vi "Img_Center_Crop.vi"(7 "Crop_CFG":T2, 8 "error in":errorcluster, 9 "Image Dest In":T1, 11 "Image Src In":T1) -> (0 "error out":errorcluster, 3 "Image Dest Out":T1)   [LabVIEW 2020]
uses:
  <vilib>/vision/Image Controls.llb/IMAQ Image.ctl
  <vilib>/Ngene/DeepLTK Anomaly Detection Addon/Toolkit/API/Controls/Crop_CFG.ctl
  <vilib>/vision/NI_Vision_Development_Module.lvlib
  <vilib>/Ngene/DeepLTK Anomaly Detection Addon/Toolkit/DeepLTK_Anomaly_Detection_Addon.lvlib
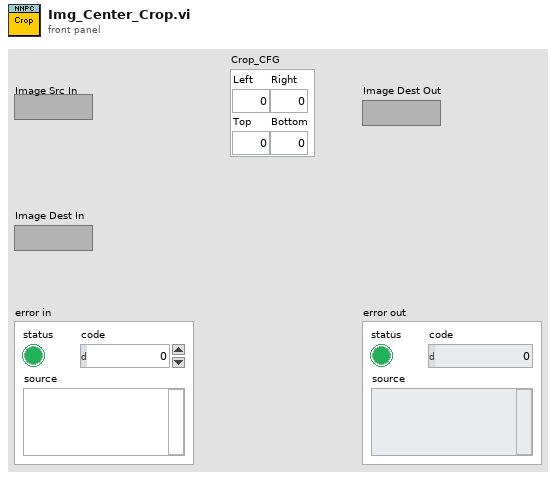
[diagram p1: front panel]
types:
  T1 = typedef "IMAQ Image.ctl" = refnum<image>
  T2 = typedef "DeepLTK_Anomaly_Detection_Addon.lvlib/Crop_CFG.ctl" = cluster{"Left":sgl, "Top":sgl, "Right":sgl, "Bottom":sgl}
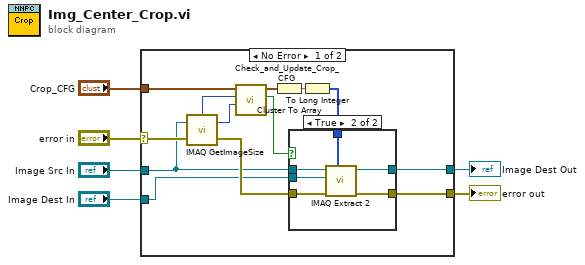
[diagram p0: block diagram]
diagram:
  n1 = case shown="No Error" "error in" {
    selector: "error in" -> [w17 w28]
    tunnel: [w19 _] -> w6
    tunnel: "Image Src In" -> [w16 _]
    tunnel: [w15 w28] -> w3
    tunnel: "Crop_CFG" -> [w14 _]
    tunnel: "Image Dest In" -> [w7 _]
    frame No Error {
      n2 = call "IMAQ GetImageSize"("Image"=w16, "error in (no error)"=w17) -> ("Y Resolution"=w12:i32, "X Resolution"=w13:i32, "error out"=w18:errorcluster)  [unwired: 2 in]
      n3 = call "Check_and_Update_Crop_CFG.vi"("Y resolution"=w12, "X resolution"=w13, "Crop_CFG_In"=w14) -> ("Valid?"=w8:bool, "Crop_CFG_Out"=w11:T2)  [unwired: 7 in]
      n4 = Cluster To Array(cluster=w11) -> (array=w10:sgl[])
      n5 = To Long Integer(number=w10) -> (32bit integer=w9:i32[])
      n6 = case shown="True" w8 {
        tunnel: [w20 w27] -> w19
        tunnel: w18 -> [w21 w26]
        tunnel: w16 -> [w20 w25]
        tunnel: [w21 w24] -> w15
        tunnel: w9 -> [_ w23]
        tunnel: w7 -> [_ w22]
        frame False {
        }
        frame True {
          n7 = call "IMAQ Extract 2"("Optional Rectangle"=w23, "error in (no error)"=w26, "Image Dst"=w22, "Image Src"=w25) -> ("error out"=w24:errorcluster, "Image Dst Out"=w27:T1)  [unwired: 6 in]
        }
      }
    }
    frame Error {
    }
  }
  "Image Dest Out" <- w6
  "error out" <- w3
